vi "Utility_Setup.vi"(6 "error in (no error)":errorcluster, 7 "Reference State (hrf)":T2, 8 "Path to Mixture file (hfmix)":path=path "C:/Program Files (x86)/National Instruments/LabVIEW 2015/user.lib/REFPROP/fluids/HMX.BNC", 9 "Mixure Cluster in":T1={"Mixture Name"="R410A", "Molecular weight (g/mol)"=72.585342534, "Critical temperature (K)"=344.507649206201, "Critical Pressure (kPa)"=4902.63149363918, "Critical Density (mol/L)"=6.3308898996459, "# Components"=2, "Fluid File Paths"=[path "C:/Program Files (x86)/National Instruments/LabVIEW 2015/user.lib/REFPROP/fluids/R32.FLD", path "C:/Program Files (x86)/National Instruments/LabVIEW 2015/user.lib/REFPROP/fluids/R125.FLD"], "Component molar fractions"=[0.697615753926276, 0.302384246073724], "Refprop Main Directory"=path "C:/Program Files (x86)/National Instruments/LabVIEW 2015/user.lib/REFPROP", "DLL Version Number"=0.0}) -> (0 "error out":errorcluster, 2 "name out":string="R410A\n*************\n1..R32         <--  0.697616 Molar fractions\ndifluoromethane    !full name                                                   ..CASN..75-10-5     \n-------------\n2..R125        <--  0.302384 Molar fractions\npentafluoroethane  !full name                                                   ..CASN..354-33-6    \n-------------\n", 3 "Mixure Cluster out":T1={"Mixture Name"="R410A", "Molecular weight (g/mol)"=72.58534253397343, "Critical temperature (K)"=344.507649206201, "Critical Pressure (kPa)"=4902.63149363918, "Critical Density (mol/L)"=6.3308898996459, "# Components"=2, "Fluid File Paths"=[path "C:/Program Files (x86)/National Instruments/LabVIEW 2015/user.lib/REFPROP/fluids/R32.FLD", path "C:/Program Files (x86)/National Instruments/LabVIEW 2015/user.lib/REFPROP/fluids/R125.FLD"], "Component molar fractions"=[0.697615753926276, 0.302384246073724], "Refprop Main Directory"=path "C:/Program Files (x86)/National Instruments/LabVIEW 2015/user.lib/REFPROP", "DLL Version Number"=9.1111})   [LabVIEW 2016]
doc: "Calls the Setupdll function in teh refprop.dll library.\n\nThis funciton must be called before any other calls to the refprop.dll.\n\nAll fluid file and mixture file paths must be absoloute paths.\n\nDeveloped by:\nGreg Sussman\nProcess Automation Corp\nwww.processauto.com\n(267)685-1249"
uses:
  Ctl/hrf_enum_d.ctl
  Ctl/Mixture Composition cluster_d.ctl
panel:
  out "herr out":string="9.1.1.11                                                                                                                                                                                                                                                       "
  out "ierr out":i32=91111
  out "wm":dbl=72.58534253397343
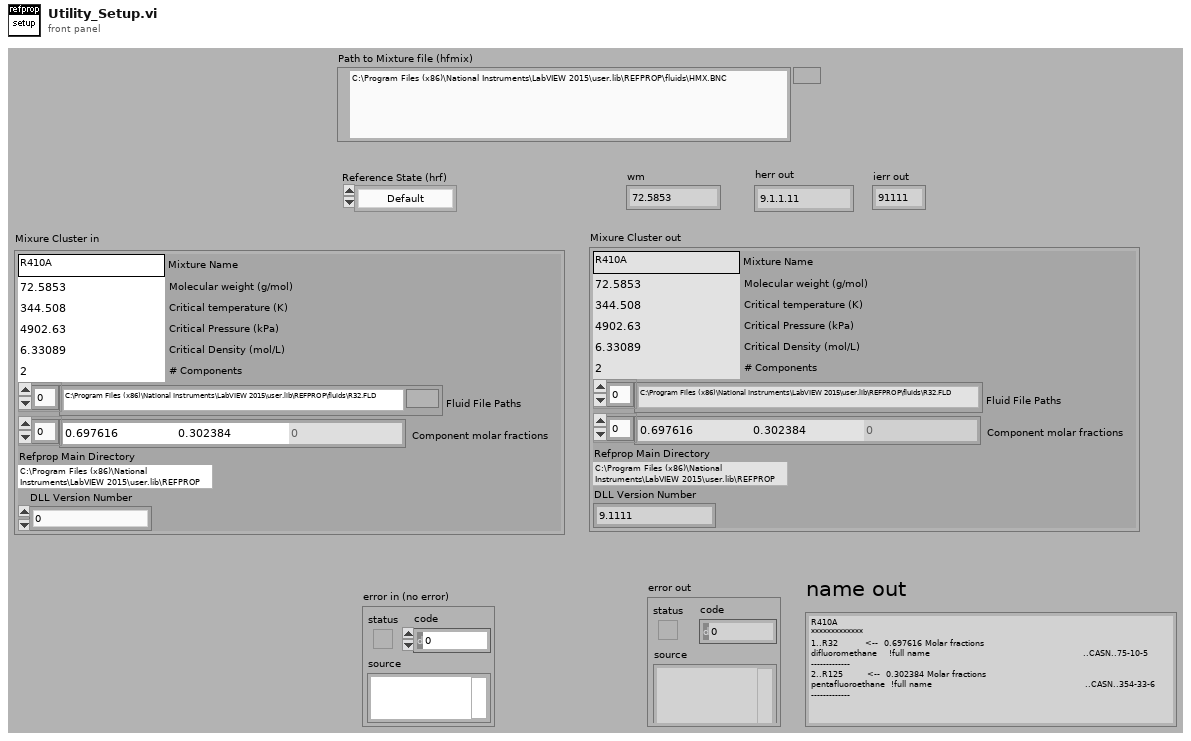
[diagram p1: front panel]
types:
  T1 = typedef "Mixture Composition cluster_d.ctl" = cluster{"Mixture Name":string, "Molecular weight (g/mol)":dbl, "Critical temperature (K)":dbl, "Critical Pressure (kPa)":dbl, "Critical Density (mol/L)":dbl, "# Components":i32, "Fluid File Paths":path[], "Component molar fractions":dbl[], "Refprop Main Directory":path, "DLL Version Number":dbl}
  T2 = typedef "hrf_enum_d.ctl" = enum16{"Default", "ASHRAE", "IIR"}
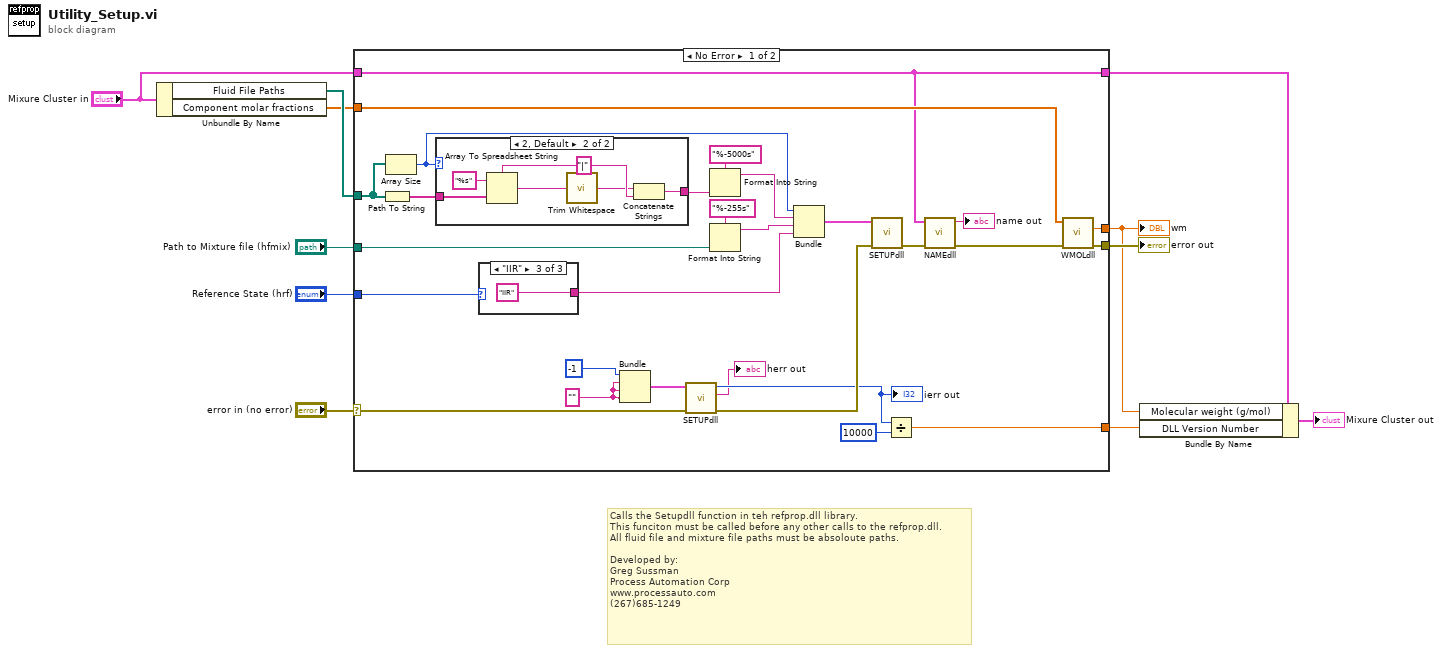
[diagram p0: block diagram]
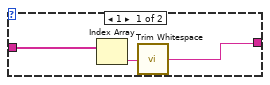
[diagram p2: hidden frame]
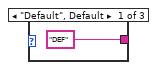
[diagram p3: hidden frame]
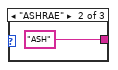
[diagram p4: hidden frame]
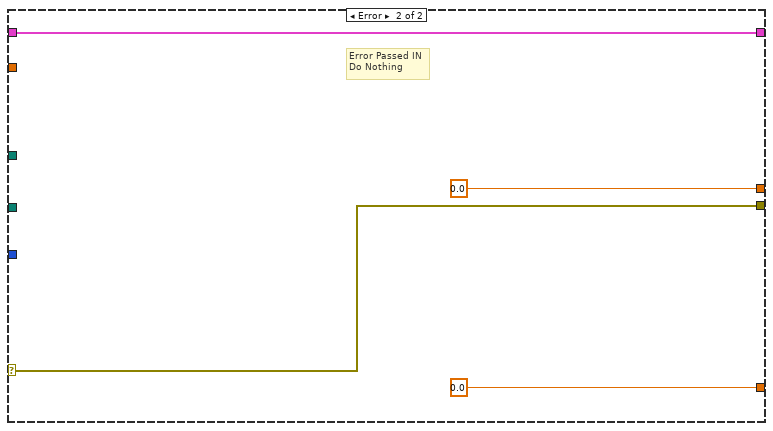
[diagram p5: hidden frame]
diagram:
  # "Calls the Setupdll function in teh refprop.dll library.\nThis funciton must be called before any other calls to the refprop.dll.\nAll fluid file and mixture file paths must be absoloute paths.\n\nDeveloped by:\nGreg Sussman\nProcess Automation Corp\nwww.processauto.com\n(267)685-1249"
  n1 = Unbundle By Name("Mixure Cluster in") -> ("Fluid File Paths"=w7:path[], "Component molar fractions"=w6:dbl[])
  n2 = case shown="No Error" "error in (no error)" {
    selector: "error in (no error)" -> [w32 w55]
    tunnel: "Path to Mixture file (hfmix)" -> [w37 _]
    tunnel: [w25 w55] -> w10
    tunnel: "Reference State (hrf)" -> [w36 _]
    tunnel: w7 -> [w33 _]
    tunnel: w6 -> [w28 _]
    tunnel: [w26 0.0 ("wm")] -> w4
    tunnel: "Mixure Cluster in" -> [w24 w53]
    tunnel: [w24 w53] -> w3
    tunnel: [w29 0.0] -> w1
    frame No Error {
      w20 = ""
      n3 = Path To String(path=w33) -> (string=w34:string[])
      n4 = Array Size(array=w33) -> (size(s)=w16:i32)
      n5 = case shown="2, Default" w16 {
        tunnel: [w40 w43] -> w35
        tunnel: w34 -> [w42 w47]
        frame 1 {
          n6 = Index Array(array=w42) -> (element=w41:string)  [unwired: 1 in]
          n7 = call <vilib>:"Trim Whitespace.vi"("string"=w41) -> ("trimmed string"=w40:string)  [unwired: 1 in]
        }
        frame 2, Default {
          w46 = "|"
          n8 = Array To Spreadsheet String(delimiter (Tab)=w46, array=w47, 3:"%s" ("format string")) -> (spreadsheet string=w45:string)
          n9 = call <vilib>:"Trim Whitespace.vi"("string"=w45) -> ("trimmed string"=w44:string)  [unwired: 1 in]
          n10 = Concatenate Strings(w44, w46) -> (w43:string)
        }
      }
      n11 = case shown="\"IIR\"" w36 {
        tunnel: ["DEF" "ASH" "IIR"] -> w13
        frame "Default", Default {
        }
        frame "ASHRAE" {
        }
        frame "IIR" {
        }
      }
      n12 = Bundle("i"=-1, w20, w20, w20) -> (w19:cluster{"i":i32, string, string, string})  [unwired: 1 in]
      n13 = call "SETUPdll.vi"("error in (no error)"=w32, "Inputs"=w19) -> ("error out"=w31:errorcluster, "herr out"=→"herr out":string, "ierr out"=w18:i32)  [unwired: 7 in]
      "ierr out" <- w18
      n14 = Format Into String(format string="%-5000s", w35) -> (resulting string=w15:string)  [unwired: 2 in, 1 out]
      n15 = Format Into String(format string="%-255s", w37) -> (resulting string=w14:string)  [unwired: 2 in, 1 out]
      n16 = Bundle(w16, w15, w14, w13) -> (w12:cluster{i32, string, string, string})  [unwired: 1 in]
      n17 = call "SETUPdll.vi"("error in (no error)"=w31, "Inputs"=w12) -> ("error out"=w22:errorcluster)  [unwired: 7 in, 2 out]
      n18 = Divide(x=w18, y=10000) -> (x/y=w29:dbl)
      n19 = call "NAMEdll.vi"("error in (no error)"=w22, "Mixure Cluster in"=w24) -> ("error out"=w27:errorcluster, "name out"=→"name out":string)  [unwired: 8 in]
      n20 = call "WMOLdll.vi"("error in (no error)"=w27, "z"=w28) -> ("error out"=w25:errorcluster, "wmm out"=w26:dbl)  [unwired: 7 in, 1 out]
    }
    frame Error {
      # "Error Passed IN\nDo Nothing"
    }
  }
  "error out" <- w10
  "wm" <- w4
  n21 = Bundle By Name(cluster=w3, "Molecular weight (g/mol)"=w4, "DLL Version Number"=w1) -> (→"Mixure Cluster out":T1)
